vi "Update.vi"(8 "error in (no error)":errorcluster, 11 "DtoA in":refnum<class "Gage 300MHz.lvclass">) -> (0 "error out":errorcluster, 3 "DtoA out":refnum<class "Gage 300MHz.lvclass">)   [LabVIEW 2014, in "Gage 300MHz.lvclass"]
doc: "Initializes a Gage 300MHz D to A to Board 0 Channel 0 by default"
uses:
  Gage 300MHz.lvclass
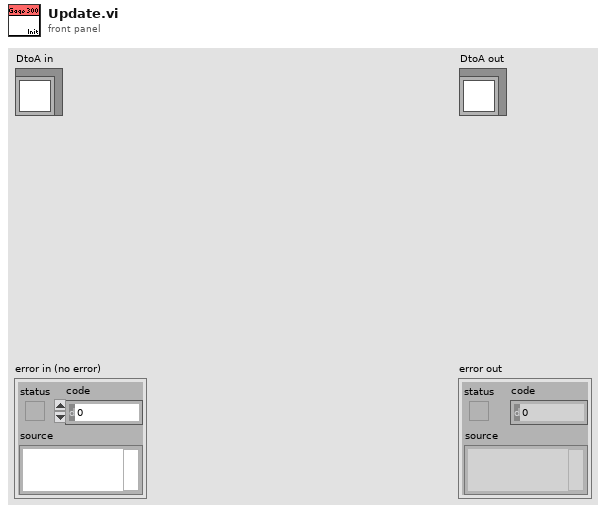
[diagram p1: front panel]
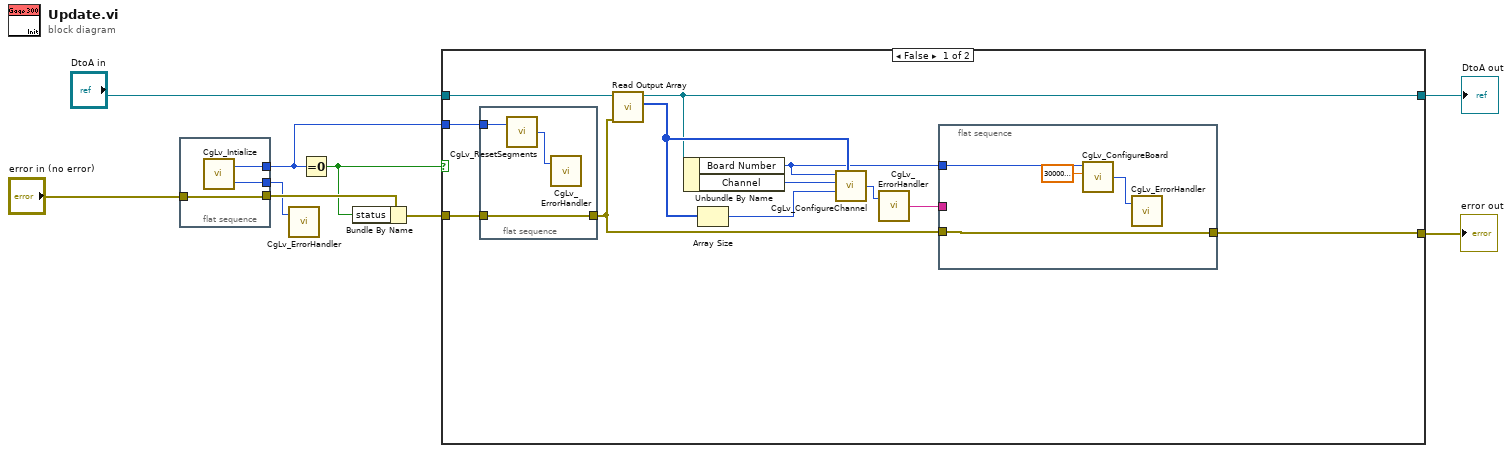
[diagram p0: block diagram]
diagram:
  n1 = flat-sequence {
    tunnel: "error in (no error)" -> [w12]
    tunnel: [w12] -> w9
    tunnel: [w11] -> w7
    tunnel: [w10] -> w5
    frame #0 {
      n2 = call "CgLv_Intialize.vi"() -> ("Error Code"=w10:i32, "Boards Found"=w11:i32)
    }
  }
  n3 = call "CgLv_ErrorHandler.vi"("Error Code"=w5) -> ()  [unwired: 1 in, 1 out]
  n4 = Equal To 0?(x=w7) -> (x = 0?=w8:bool)
  n5 = Bundle By Name(cluster=w9, "status"=w8) -> (w6:errorcluster)
  n6 = case shown="False" w8 {
    tunnel: w7 -> [w24 _]
    tunnel: w6 -> [w22 w33]
    tunnel: "DtoA in" -> [w23 w32]
    tunnel: [w14 w33] -> w3
    tunnel: [w13 w32] -> w4
    frame False {
      n7 = flat-sequence {
        tunnel: w24 -> [w31]
        tunnel: w22 -> [w30]
        tunnel: [w30] -> w16
        frame #0 {
          n8 = call "CgLv_ResetSegments.vi"("Board Number (0)"=w31) -> ("Error Code"=w29:i32)  [unwired: 1 in]
          n9 = call "CgLv_ErrorHandler.vi"("Error Code"=w29) -> ()  [unwired: 1 in, 1 out]
        }
      }
      n10 = call-dynamic "Read Output Array.vi"("error in (no error)"=w16, "DtoA in"=w23) -> ("Output Array"=w19:u16[], "DtoA out"=w13:refnum<class "Gage 300MHz.lvclass">)  [unwired: 7 in, 1 out]
      n11 = Unbundle By Name(w13) -> ("Board Number"=w15:u32, "Channel"=w21:u32)
      n12 = Array Size(array=w19) -> (size(s)=w20:i32)
      n13 = call "CgLv_ConfigureChannel.vi"("Board Number (0)"=w15, "Channel Number (1)"=w21, "Buffer Length (1024)"=w20, "Buffer"=w19) -> ("Error Code"=w18:i32)  [unwired: 1 in]
      n14 = call "CgLv_ErrorHandler.vi"("Error Code"=w18) -> ("Error String"=w17:string)  [unwired: 1 in]
      n15 = flat-sequence {
        tunnel: w17 -> [_]
        tunnel: w16 -> [w25]
        tunnel: w15 -> [w28]
        tunnel: [w25] -> w14
        frame #0 {
          n16 = call "CgLv_ConfigureBoard.vi"("Conversion Rate (150 MHz)"=sgl 300000000.0, "Board Number (0)"=w28) -> ("Error Code"=w26:i32)  [unwired: 2 in]
          n17 = call "CgLv_ErrorHandler.vi"("Error Code"=w26) -> ()  [unwired: 1 in, 1 out]
        }
      }
    }
    frame True {
    }
  }
  "error out" <- w3
  "DtoA out" <- w4
